vi "Set Output Values.vi"(8 "error in (no error)":errorcluster, 11 "Spectrum Recorder in":refnum<class "Spectrum Recorder too.lvclass">) -> (0 "error out":errorcluster, 3 "Spectrum Recorder out":refnum<class "Spectrum Recorder too.lvclass">)   [LabVIEW 2016, in "Spectrum Recorder too.lvclass"]
uses:
  Spectrum Recorder too.lvclass
  Spectrum Recorder too.lvclass/Spectrum Recorder too.ctl
  Read Spectrum Recorder Configuration.vi
  Read RP transceiver.vi
  Write RP transceiver.vi
  NHMFL_Core/Libraries/Red Pitaya/RP Core/RP Transceiver/RP Transceiver.lvclass
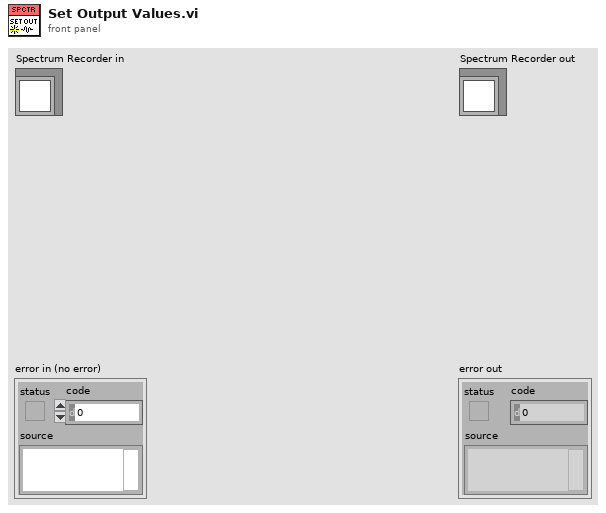
[diagram p1: front panel]
types:
  T1 = typedef "Spectrum Recorder Configuration.ctl" = cluster{"Start":dbl, "End":dbl, "Duration":dbl, "Filter time constant":dbl, "Repeat (-1: forever)":i32, "Update rate":dbl, "Data storage folder":path}
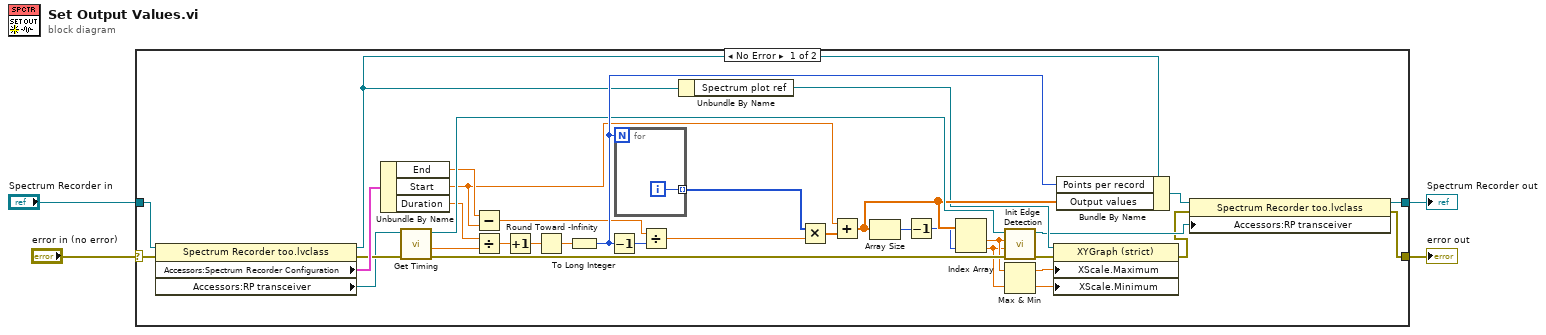
[diagram p0: block diagram]
diagram:
  n1 = case shown="No Error" "error in (no error)" {
    selector: "error in (no error)" -> [w13 w42]
    tunnel: [w5 w42] -> w3
    tunnel: [w8 w41] -> w1
    tunnel: "Spectrum Recorder in" -> [w16 w41]
    frame No Error {
      n2 = property class="Spectrum Recorder too.lvclass"(reference=w16, error in=w13) -> (reference out=w15:refnum<class "Spectrum Recorder too.lvclass">, error out=w14:errorcluster, "Accessors:Spectrum Recorder Configuration"=w17:T1, "Accessors:RP transceiver"=w9:refnum<class "RP Transceiver.lvclass">)
      n3 = Unbundle By Name(w17) -> ("End"=w12:dbl, "Start"=w11:dbl, "Duration"=w10:dbl)
      n4 = call-dynamic "Get Timing.vi"("error in (no error)"=w14, "RP Transceiver in"=w9) -> ("error out"=w28:errorcluster, "dt"=w30:dbl, "RP Transceiver out"=w27:refnum<class "RP Transceiver.lvclass">)  [unwired: 5 in, 2 out]
      n5 = Subtract(x=w12, y=w11) -> (x-y=w35:dbl)
      n6 = Divide(x=w10, y=w30) -> (x/y=w33:dbl)
      n7 = Increment(x=w33) -> (x+1=w32:dbl)
      n8 = Round Toward -Infinity(1:w32) -> (0:w31:dbl)
      n9 = To Long Integer(number=w31) -> (32bit integer=w36:i32)
      n10 = Decrement(x=w36) -> (x-1=w34:i32)
      n11 = for {
        N: w36 -> [_]
        tunnel: [w40] -> w38 mode=indexing
        i -> [w40]
      }
      n12 = Divide(x=w35, y=w34) -> (x/y=w37:dbl)
      n13 = Unbundle By Name(w15) -> ("Spectrum plot ref"=w23:refnum<vi>)
      n14 = Multiply(x=w38, y=w37) -> (x*y=w39:dbl[])
      n15 = Add(x=w11, y=w39) -> (x+y=w26:dbl[])
      n16 = Array Size(array=w26) -> (size(s)=w25:i32)
      n17 = Decrement(x=w25) -> (x-1=w24:i32)
      n18 = Index Array(array=w26, index #2=w24) -> (element #1=w21:dbl, element #2=w20:dbl)  [unwired: 1 in]
      n19 = call-dynamic "Init Edge Detection.vi"("error in (no error)"=w28, "Last output"=w20, "First output"=w21, "RP Transceiver in"=w27) -> ("error out"=w22:errorcluster, "RP Transceiver out"=w7:refnum<class "RP Transceiver.lvclass">)  [unwired: 6 in]
      n20 = Max & Min(x=w21, y=w20) -> (max(x,y)=w19:dbl, min(x,y)=w18:dbl)
      n21 = property class="XYGraph (strict)"(reference=w23, error in=w22, "XScale.Maximum"=w19, "XScale.Minimum"=w18) -> (error out=w6:errorcluster)  [unwired: 1 out]
      n22 = Bundle By Name(cluster=w15, "Points per record"=w36, "Output values"=w26) -> (w29:refnum<class "Spectrum Recorder too.lvclass">)
      n23 = property class="Spectrum Recorder too.lvclass"(reference=w29, error in=w6, "Accessors:RP transceiver"=w7) -> (reference out=w8:refnum<class "Spectrum Recorder too.lvclass">, error out=w5:errorcluster)
    }
    frame Error {
    }
  }
  "error out" <- w3
  "Spectrum Recorder out" <- w1
